vi "ABB Select configure.vi"() -> ()   [LabVIEW 2017]
panel:
  in  "VT&CT Ratios":bool
  in  "Efficiencies":bool
  in  "Test Instruments":bool
  in  "Test personel":bool
  in  "Bearing Inspection":bool
  in  "Noise Test":bool
  in  "Report":bool
  in  "Bearing run":bool
  in  "Locked rotor":bool
  in  "No Load":bool
  in  "Temperatures":bool
  in  "Heat Run":bool
  in  "System":bool
  in  "Exit":bool
  # "Configure"
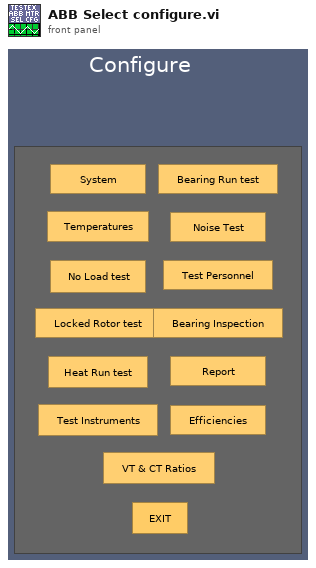
[diagram p1: front panel]
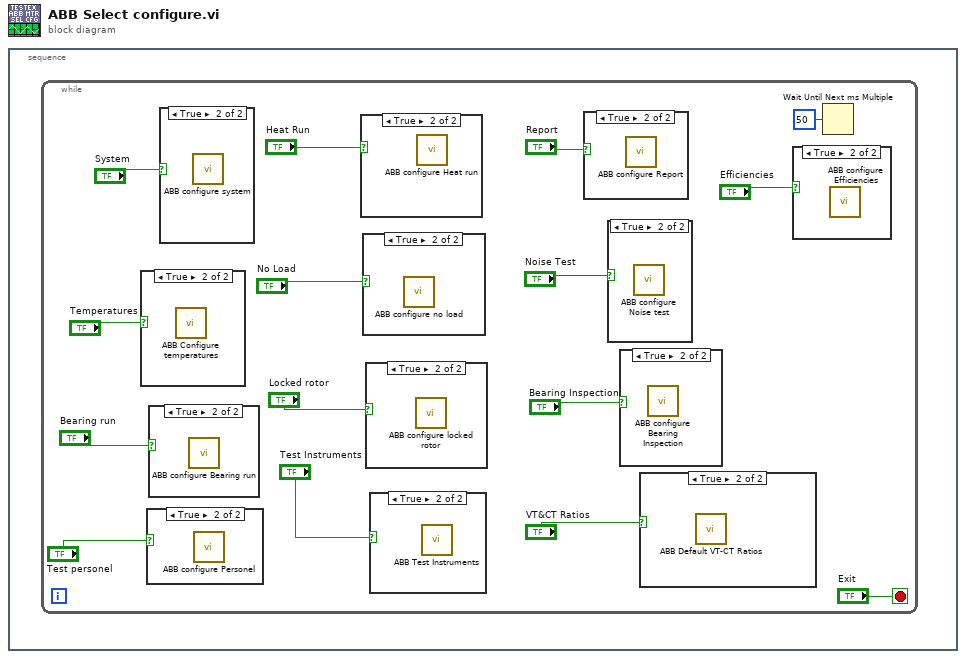
[diagram p0: block diagram]
diagram:
  n1 = stacked-sequence {
    frame #0 {
      n2 = while {
        stop <- "Exit" stop-if-true
        n3 = case shown="True" "Temperatures" {
          frame False {
          }
          frame True {
            n4 = call "ABB Configure temperatures.vi"() -> ()  [unwired: 1 in]
          }
        }
        n5 = case shown="True" "Test personel" {
          frame False {
          }
          frame True {
            n6 = call "ABB configure Personel.vi"() -> ()  [unwired: 1 in]
          }
        }
        n7 = case shown="True" "Bearing run" {
          frame False {
          }
          frame True {
            n8 = call "ABB configure Bearing run.vi"() -> ()  [unwired: 1 in]
          }
        }
        n9 = case shown="True" "System" {
          frame False {
          }
          frame True {
            n10 = call "ABB configure system.vi"() -> ()  [unwired: 1 in]
          }
        }
        n11 = case shown="True" "Heat Run" {
          frame False {
          }
          frame True {
            n12 = call "ABB configure Heat run.vi"() -> ()  [unwired: 1 in]
          }
        }
        n13 = case shown="True" "No Load" {
          frame False {
          }
          frame True {
            n14 = call "ABB configure no load.vi"() -> ()  [unwired: 1 in]
          }
        }
        n15 = case shown="True" "Locked rotor" {
          frame False {
          }
          frame True {
            n16 = call "ABB configure locked rotor.vi"() -> ()  [unwired: 1 in]
          }
        }
        n17 = case shown="True" "Test Instruments" {
          frame False {
          }
          frame True {
            n18 = call "ABB Test Instruments.vi"() -> ()  [unwired: 1 in]
          }
        }
        n19 = case shown="True" "Report" {
          frame False {
          }
          frame True {
            n20 = call "ABB configure Report.vi"() -> ()  [unwired: 1 in]
          }
        }
        n21 = case shown="True" "Noise Test" {
          frame False {
          }
          frame True {
            n22 = call "ABB configure Noise test.vi"() -> ()  [unwired: 1 in]
          }
        }
        n23 = case shown="True" "Bearing Inspection" {
          frame False {
          }
          frame True {
            n24 = call "ABB configure Bearing Inspection.vi"() -> ()  [unwired: 1 in]
          }
        }
        n25 = case shown="True" "VT&CT Ratios" {
          frame False {
          }
          frame True {
            n26 = call "ABB Default VT-CT Ratios.vi"() -> ()  [unwired: 12 in]
          }
        }
        n27 = case shown="True" "Efficiencies" {
          frame False {
          }
          frame True {
            n28 = call "ABB configure Efficiencies.vi"() -> ()  [unwired: 1 in]
          }
        }
        n29 = Wait Until Next ms Multiple(millisecond multiple=u32 50) -> ()  [unwired: 1 out]
      }
    }
  }
